vi "Agilent_GPIB_FSM.vi"(7 "error in":errorcluster, 8 "MEAS":refnum<queue>, 9 "GPIB":string, 10 "commands":refnum<queue>) -> ()   [LabVIEW 2021, in "GPIB_UART.lvlib"]
uses:
  GPIB_UART.lvlib
panel:
  out "OUTPUT CURRENT [mA]":dbl
  out "LIMIT Current":dbl
  out "error out":errorcluster
  in  "Stop Button":bool
  out "state_and_args":string
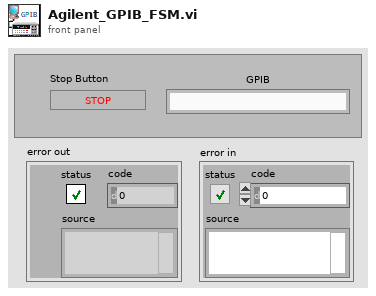
[diagram p1: front panel]
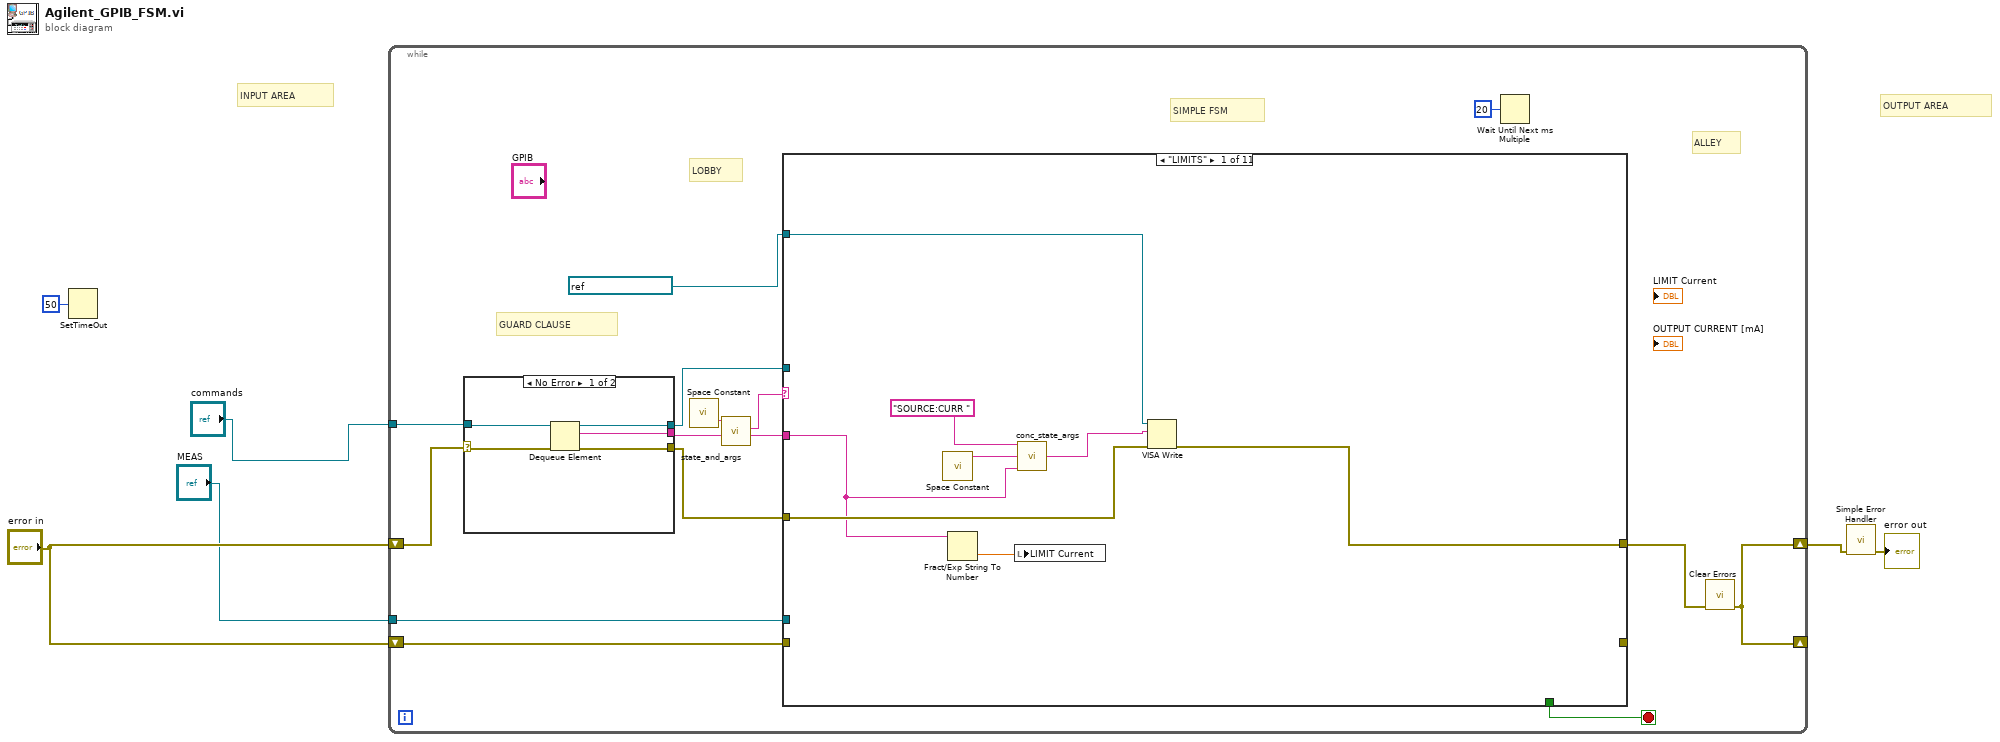
[diagram p0: block diagram]
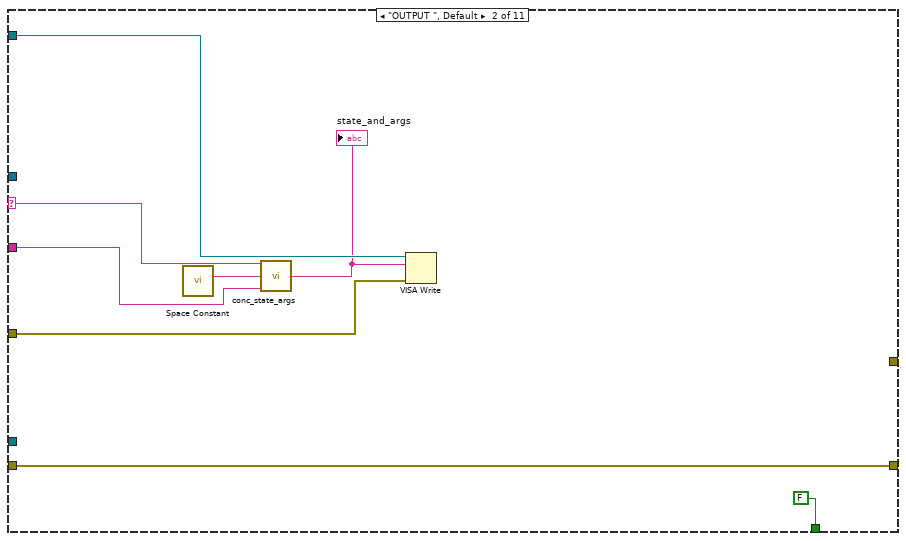
[diagram p2: hidden frame]
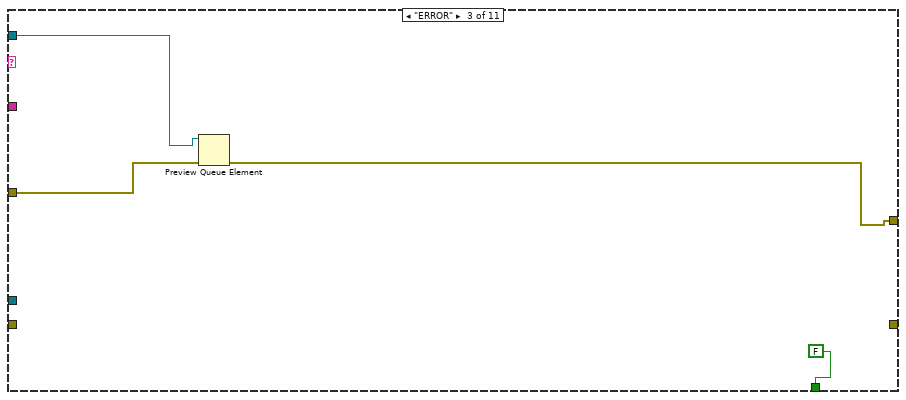
[diagram p3: hidden frame]
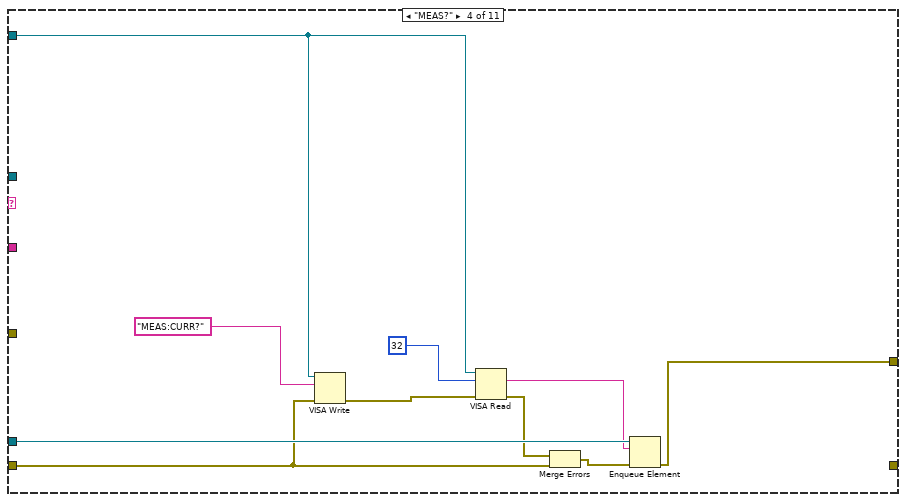
[diagram p4: hidden frame]
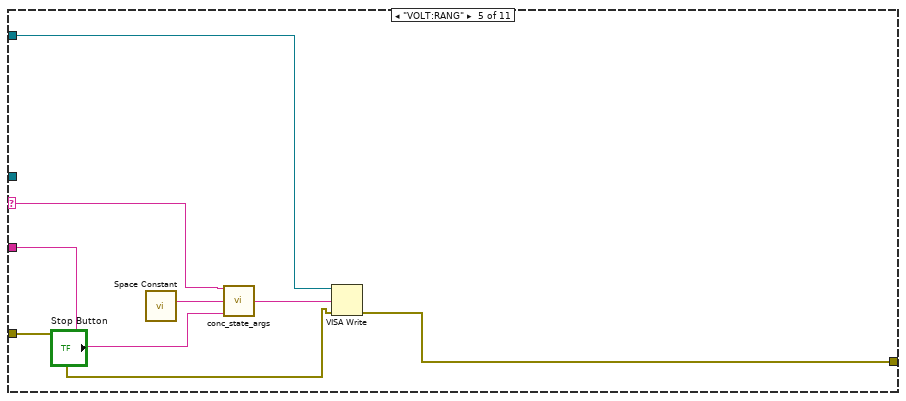
[diagram p5: hidden frame]
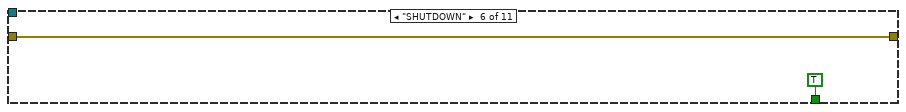
[diagram p6: hidden frame]
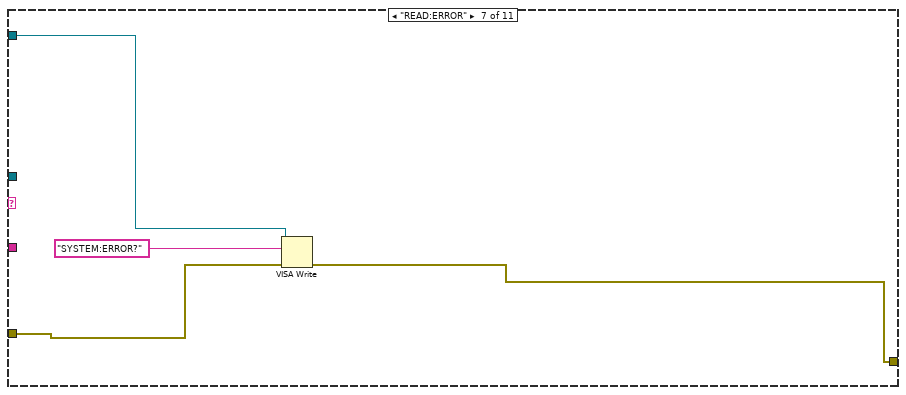
[diagram p7: hidden frame]
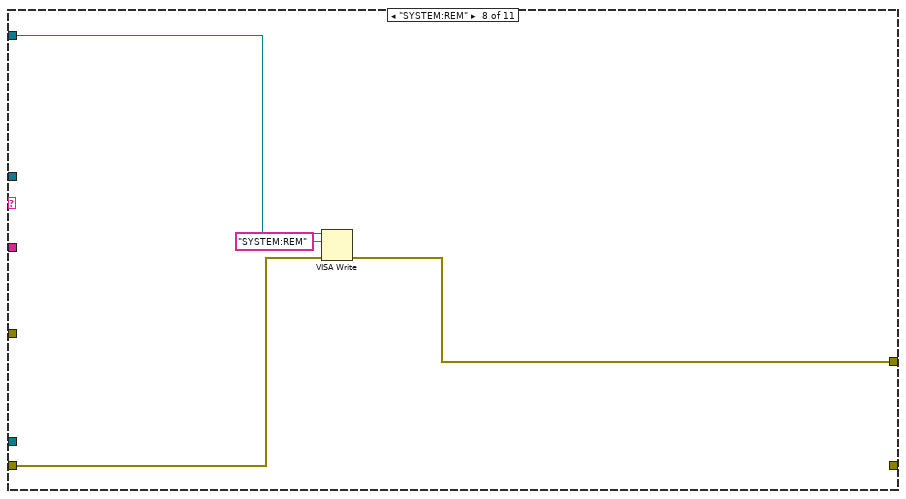
[diagram p8: hidden frame]
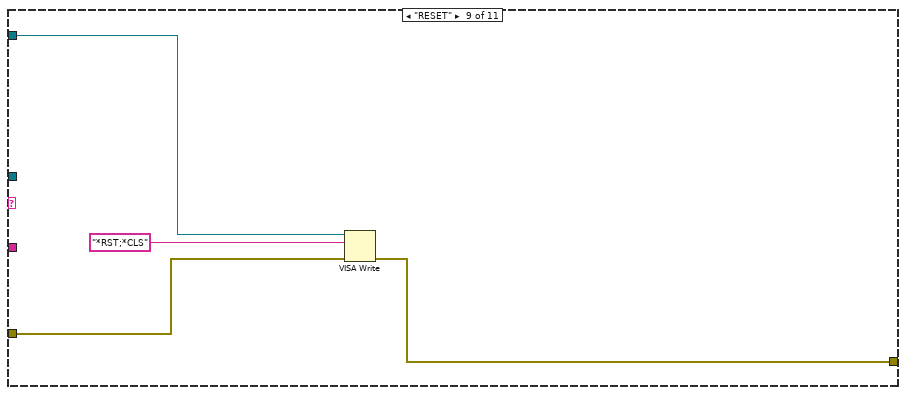
[diagram p9: hidden frame]
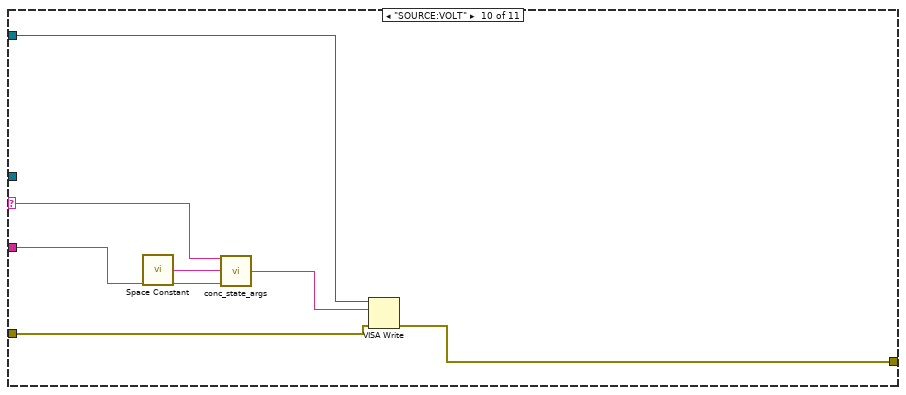
[diagram p10: hidden frame]
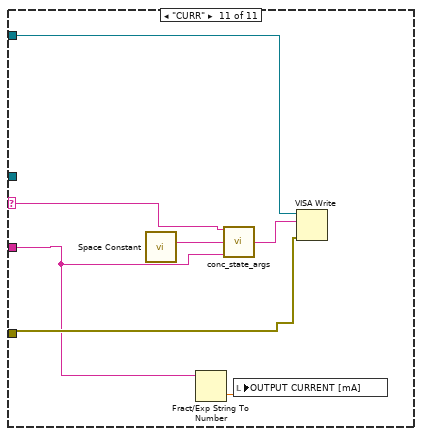
[diagram p11: hidden frame]
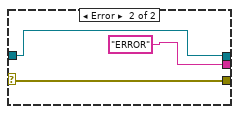
[diagram p12: hidden frame]
diagram:
  # "OUTPUT AREA"
  # "INPUT AREA"
  n1 = SetTimeOut(1:50 ("new timeout (10000)")) -> ()  [unwired: 1 out]
  n2 = while {
    tunnel: "commands" -> [w20]
    shift-right: [w7] -> w5
    shift-left: "error in" -> [w21]
    shift-right: [w7] -> _
    shift-left: "error in" -> [w12]
    tunnel: "MEAS" -> [w11]
    stop <- w13 stop-if-true
    # "SIMPLE FSM"
    # "ALLEY"
    # "LOBBY"
    # "GUARD CLAUSE"
    n3 = case shown="No Error" w21 {
      selector: w21 -> [w90 w92]
      tunnel: w20 -> [w91 w93]
      tunnel: [w89 w93] -> w14
      tunnel: [w88 w92] -> w16
      tunnel: [w87 "ERROR"] -> w19
      frame No Error {
        n4 = Dequeue Element(queue=w91, error in (no error)=w90) -> (queue out=w89:refnum<queue>, element=w87:string, error out=w88:errorcluster)  [unwired: 1 in, 1 out]
      }
      frame Error {
      }
    }
    n5 = call <vilib>:"Space Constant.vi"() -> ("String"=w18:string)
    n6 = call "state_and_args.vi"("String"=w19, "DELIMITER (:)"=w18) -> ("Arguments"=w15:string, "State"=w17:string)  [unwired: 8 in]
    n7 = case shown="\"LIMITS\"" w17 {
      selector: w17 -> [_ w35 _ _ w55 _ _ _ _ w78 w84]
      tunnel: w16 -> [w26 w34 w40 _ w54 _ w62 _ w70 w74 w83]
      tunnel: w15 -> [w23 w37 _ _ w56 _ _ _ _ w79 w81]
      tunnel: refnum<visa-resource-name> "GPIB0::1::INSTR" ("VISA resource name") -> [w27 w36 _ w50 w58 _ w64 w68 w72 w76 w86]
      tunnel: [w25 _ w39 w46 w53 _ w61 w65 w69 w73 _] -> w8
      tunnel: w14 -> [_ _ w41 _ _ _ _ _ _ _ _]
      tunnel: [_ FALSE FALSE _ _ TRUE _ _ _ _ _] -> w13
      tunnel: w12 -> [_ w31 _ w45 _ w59 _ w66 _ _ _]
      tunnel: w11 -> [_ _ _ w47 _ _ _ _ _ _ _]
      tunnel: [_ w31 _ _ _ w59 _ _ _ _ _] -> _
      frame "LIMITS" {
        n8 = call <vilib>:"Space Constant.vi"() -> ("String"=w29:string)
        n9 = Fract/Exp String To Number(string=w23) -> (number=w24:dbl)  [unwired: 3 in, 1 out]
        n10 = local write "LIMIT Current"(w24) -> ()
        n11 = call "conc_state_args.vi"("State"="SOURCE:CURR ", "DELIMITER (:)"=w29, "Args"=w23) -> ("state_and_args"=w22:string)  [unwired: 12 in]
        n12 = VISA Write(VISA resource name=w27, write buffer=w22, error in (no error)=w26) -> (error out=w25:errorcluster)  [unwired: 2 out]
      }
      frame "OUTPUT ", Default {
        n13 = call <vilib>:"Space Constant.vi"() -> ("String"=w33:string)
        n14 = call "conc_state_args.vi"("State"=w35, "DELIMITER (:)"=w33, "Args"=w37) -> ("state_and_args"=w30:string)  [unwired: 12 in]
        "state_and_args" <- w30
        n15 = VISA Write(VISA resource name=w36, write buffer=w30, error in (no error)=w34) -> ()  [unwired: 3 out]
      }
      frame "ERROR" {
        n16 = Preview Queue Element(queue=w41, error in (no error)=w40) -> (error out=w39:errorcluster)  [unwired: 1 in, 3 out]
      }
      frame "MEAS?" {
        n17 = VISA Write(VISA resource name=w50, write buffer="MEAS:CURR?", error in (no error)=w45) -> (error out=w51:errorcluster)  [unwired: 2 out]
        n18 = VISA Read(VISA resource name=w50, byte count=32, error in (no error)=w51) -> (read buffer=w42:string, error out=w43:errorcluster)  [unwired: 2 out]
        n19 = Merge Errors(w43, w45) -> (w48:errorcluster)
        n20 = Enqueue Element(queue=w47, element=w42, error in (no error)=w48) -> (error out=w46:errorcluster)  [unwired: 1 in, 2 out]
      }
      frame "VOLT:RANG" {
        n21 = call <vilib>:"Space Constant.vi"() -> ("String"=w57:string)
        n22 = call "conc_state_args.vi"("State"=w55, "DELIMITER (:)"=w57, "Args"=w56) -> ("state_and_args"=w52:string)  [unwired: 12 in]
        n23 = VISA Write(VISA resource name=w58, write buffer=w52, error in (no error)=w54) -> (error out=w53:errorcluster)  [unwired: 2 out]
      }
      frame "SHUTDOWN" {
      }
      frame "READ:ERROR" {
        n24 = VISA Write(VISA resource name=w64, write buffer="SYSTEM:ERROR?" ("data"), error in (no error)=w62) -> (error out=w61:errorcluster)  [unwired: 2 out]
      }
      frame "SYSTEM:REM" {
        n25 = VISA Write(VISA resource name=w68, write buffer="SYSTEM:REM" ("data"), error in (no error)=w66) -> (error out=w65:errorcluster)  [unwired: 2 out]
      }
      frame "RESET" {
        n26 = VISA Write(VISA resource name=w72, write buffer="*RST;*CLS" ("data"), error in (no error)=w70) -> (error out=w69:errorcluster)  [unwired: 2 out]
      }
      frame "SOURCE:VOLT" {
        n27 = call <vilib>:"Space Constant.vi"() -> ("String"=w77:string)
        n28 = call "conc_state_args.vi"("State"=w78, "DELIMITER (:)"=w77, "Args"=w79) -> ("state_and_args"=w75:string)  [unwired: 12 in]
        n29 = VISA Write(VISA resource name=w76, write buffer=w75, error in (no error)=w74) -> (error out=w73:errorcluster)  [unwired: 2 out]
      }
      frame "CURR" {
        n30 = call <vilib>:"Space Constant.vi"() -> ("String"=w85:string)
        n31 = Fract/Exp String To Number(string=w81) -> (number=w82:dbl)  [unwired: 3 in, 1 out]
        n32 = call "conc_state_args.vi"("State"=w84, "DELIMITER (:)"=w85, "Args"=w81) -> ("state_and_args"=w80:string)  [unwired: 12 in]
        n33 = local write "OUTPUT CURRENT [mA]"(w82) -> ()
        n34 = VISA Write(VISA resource name=w86, write buffer=w80, error in (no error)=w83) -> ()  [unwired: 3 out]
      }
    }
    n35 = Wait Until Next ms Multiple(millisecond multiple=u32 20) -> ()  [unwired: 1 out]
    n36 = call <vilib>:"Clear Errors.vi"("error in (no error)"=w8) -> ("error out"=w7:errorcluster)  [unwired: 5 in, 1 out]
  }
  n37 = call <vilib>:"Simple Error Handler.vi"("error in (no error)"=w5) -> ("error out"=→"error out":errorcluster)  [unwired: 4 in, 4 out]
